vi "ttlPulser.vi"() -> ()   [LabVIEW 2019]
uses:
  <vilib>/DAQmx/write.llb/DAQmx Write (Digital Bool 1Line 1Point).vi
  <vilib>/DAQmx/create/channels.llb/DAQmx Create Channel (DO-Digital Output).vi
  <vilib>/DAQmx/miscellaneous.llb/DAQmx Fill In Error Info.vi
panel:
  in  "stop":bool
  out "error out":errorcluster
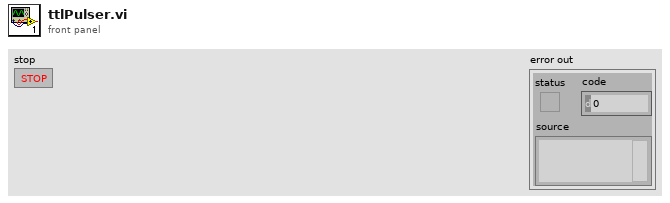
[diagram p1: front panel]
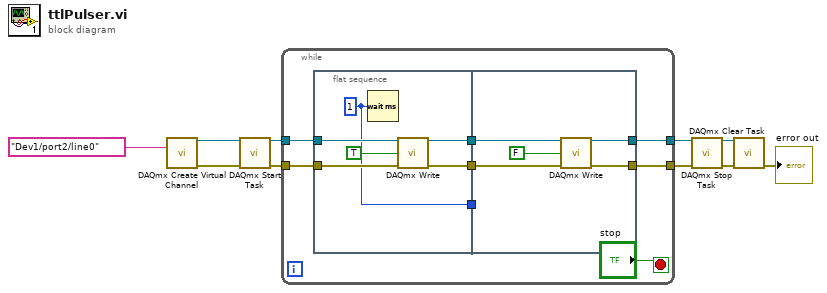
[diagram p0: block diagram]
diagram:
  n1 = call-poly <vilib>:"DAQmx Create Virtual Channel.vi"("lines"=tag "Dev1/port2/line0") -> ("task out"=w9:refnum<k21>, "error out"=w8:errorcluster)  [unwired: 13 in]
  n2 = call <vilib>:"DAQmx Start Task.vi"("task/channels in"=w9, "error in"=w8) -> ("task out"=w7:refnum<k21>, "error out"=w6:errorcluster)  [unwired: 12 in]
  n3 = while {
    tunnel: w7 -> [w16]
    tunnel: w6 -> [w15]
    tunnel: [w14] -> w5
    tunnel: [w13] -> w4
    stop <- "stop" stop-if-true
    n4 = flat-sequence {
      tunnel: [w24] -> w18
      tunnel: [w23] -> w17
      tunnel: w16 -> [w21]
      tunnel: w15 -> [w20]
      tunnel: [w19] -> w11
      tunnel: w18 -> [w29]
      tunnel: w17 -> [w28]
      tunnel: [w26] -> w14
      tunnel: [w25] -> w13
      tunnel: w11 -> [_]
      frame #0 {
        w19 = u32 1 ("milliseconds to wait")
        n5 = Wait (ms)(milliseconds to wait=w19) -> ()  [unwired: 1 out]
        n6 = call-poly <vilib>:"DAQmx Write.vi"("task/channels in"=w21, "data"=TRUE, "error in"=w20) -> ("task out"=w24:refnum<k21>, "error out"=w23:errorcluster)  [unwired: 10 in, 1 out]
      }
      frame #1 {
        n7 = call-poly <vilib>:"DAQmx Write.vi"("task/channels in"=w29, "data"=FALSE, "error in"=w28) -> ("task out"=w26:refnum<k21>, "error out"=w25:errorcluster)  [unwired: 10 in, 1 out]
      }
    }
  }
  n8 = call <vilib>:"DAQmx Stop Task.vi"("task/channels in"=w5, "error in"=w4) -> ("task out"=w3:refnum<k21>, "error out"=w2:errorcluster)  [unwired: 12 in]
  n9 = call <vilib>:"DAQmx Clear Task.vi"("task in"=w3, "error in"=w2) -> ("error out"=→"error out":errorcluster)  [unwired: 13 in]
